vi "SW Arch draft.vi"() -> ()   [LabVIEW 2009]
panel:
  out "Main State":string
  out "VFH cluster":cluster{"VFH Message":string, "VFH Data":i32[]}={"VFH Message"="1000", "VFH Data"=[]}
  in  "Motor Message":string
  out "Sensor cluster":T1
  out "Motor Queue":refnum<queue>
  out "VFH Queue":refnum<queue>
  out "Communication Queue":refnum<queue>
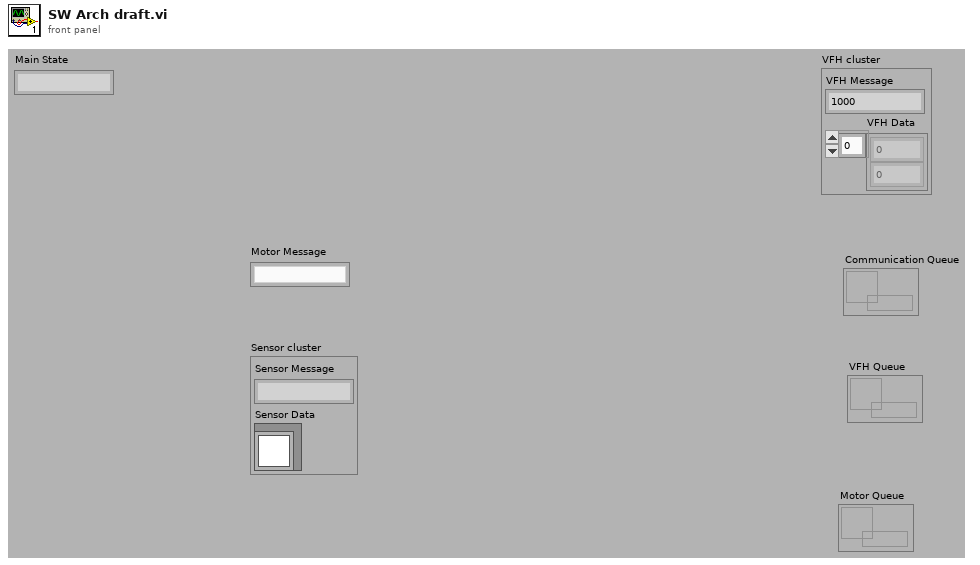
[diagram p1: front panel]
types:
  T1 = cluster{"Sensor Message":string, "Sensor Data":refnum<class>}
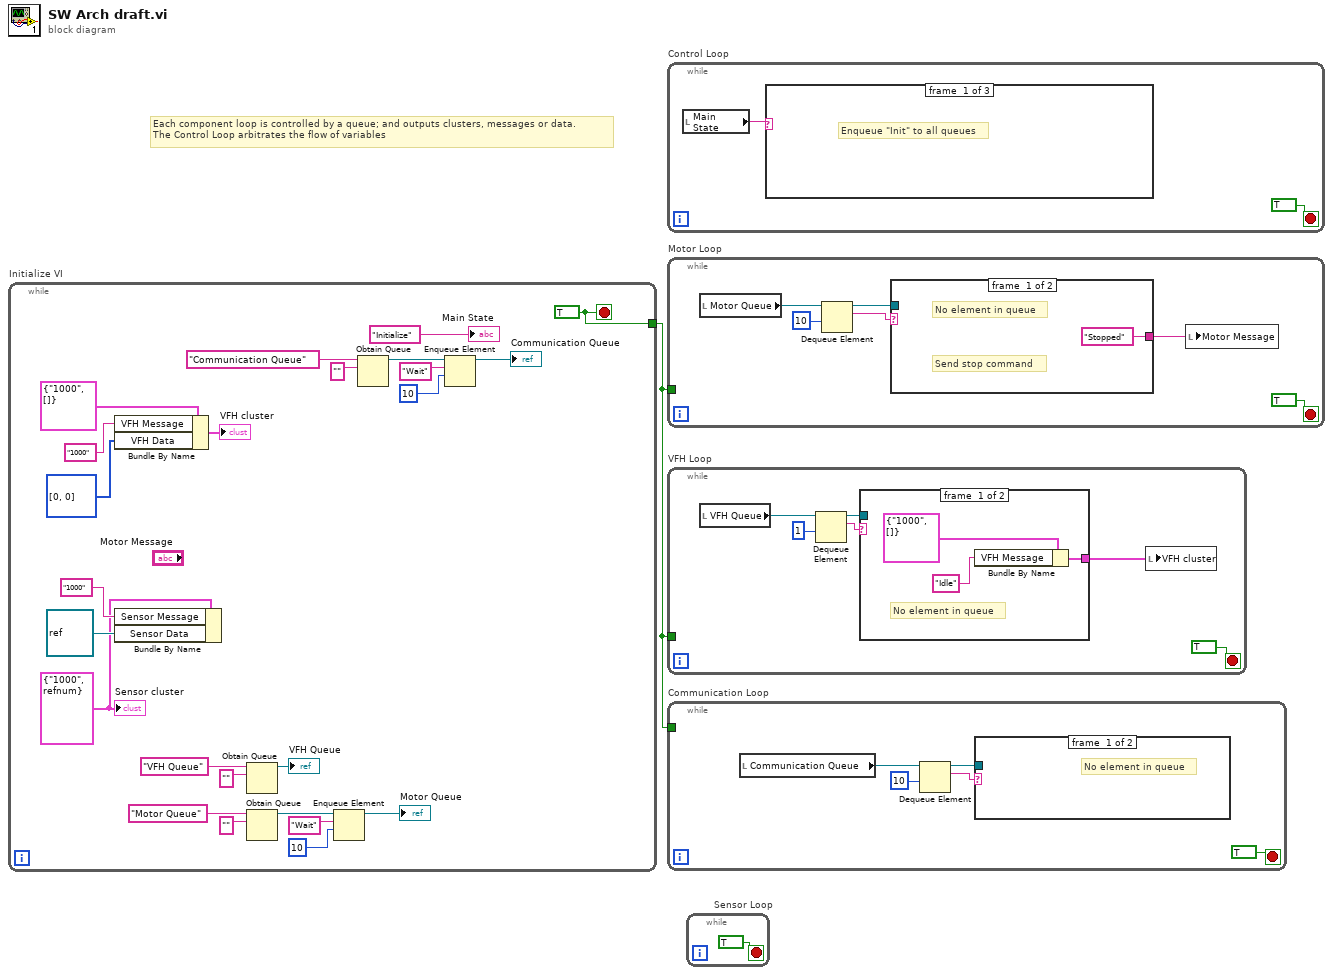
[diagram p0: block diagram]
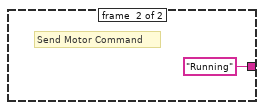
[diagram p4: hidden frame]
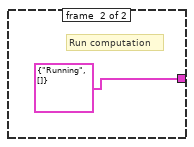
[diagram p5: hidden frame]
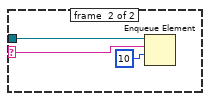
[diagram p6: hidden frame]
diagram:
  # "Each component loop is controlled by a queue; and outputs clusters, messages or data.\nThe Control Loop arbitrates the flow of variables"
  n1 = while "Initialize VI" {
    tunnel: [w10] -> w1
    stop <- w10 stop-if-true
    w5 = T1 {"Sensor Message"="1000", "Sensor Data"=refnum} ("Sensor cluster")
    w10 = TRUE
    n2 = Bundle By Name(cluster=cluster{"VFH Message":string, "VFH Data":i32[]} {"VFH Message"="1000", "VFH Data"=[]} ("VFH cluster"), "VFH Message"="1000", "VFH Data"=i32[] [0, 0]) -> (→"VFH cluster":cluster{"VFH Message":string, "VFH Data":i32[]})
    n3 = Bundle By Name(cluster=w5, "Sensor Message"="1000" ("VFH Message"), "Sensor Data"=refnum<class> refnum) -> ()  [unwired: 1 out]
    n4 = Obtain Queue(name (unnamed)="VFH Queue", element data type="" ("name (unnamed)")) -> (queue out=→"VFH Queue":refnum<queue>)  [unwired: 3 in, 2 out]
    n5 = Obtain Queue(name (unnamed)="Motor Queue", element data type="" ("name (unnamed)")) -> (queue out=w17:refnum<queue>)  [unwired: 3 in, 2 out]
    n6 = Enqueue Element(queue=w17, element="Wait", timeout in ms (-1)=10) -> (queue out=→"Motor Queue":refnum<queue>)  [unwired: 1 in, 2 out]
    n7 = Obtain Queue(name (unnamed)="Communication Queue", element data type="" ("name (unnamed)")) -> (queue out=w25:refnum<queue>)  [unwired: 3 in, 2 out]
    n8 = Enqueue Element(queue=w25, element="Wait", timeout in ms (-1)=10) -> (queue out=→"Communication Queue":refnum<queue>)  [unwired: 1 in, 2 out]
    "Sensor cluster" <- w5
    "Main State" <- "Initialize" ("Main State")
  }
  n9 = while "Control Loop" {
    stop <- TRUE stop-if-true
    n10 = local read "Main State"() -> (w26:string)
    n11 = case shown="\"RC Run\"" w26 {
      frame #0 {
        # "Enqueue \"Init\" to all queues"
      }
      frame #1 {
        # "Run Sensor\nRun VFH on new SICK data\nSensor Data -> VFH\nVFH Data -> Motor"
      }
      frame #2 {
        # "Communication Data -> Motor"
      }
    }
  }
  n12 = while "Motor Loop" {
    tunnel: w1 -> [_]
    stop <- TRUE stop-if-true
    n13 = local read "Motor Queue"() -> (w33:refnum<queue>)
    n14 = Dequeue Element(queue=w33, timeout in ms (-1)=10) -> (queue out=w30:refnum<queue>, element=w32:string)  [unwired: 1 in, 2 out]
    n15 = case shown="\"Run\"" w32 {
      tunnel: w30 -> [_ _]
      tunnel: ["Stopped" ("Motor Message") "Running" ("Motor Message")] -> w28
      frame #0 {
        # "Send stop command"
        # "No element in queue"
      }
      frame #1 {
        # "Send Motor Command"
      }
    }
    n16 = local write "Motor Message"(w28) -> ()
  }
  n17 = while "VFH Loop" {
    tunnel: w1 -> [_]
    stop <- TRUE stop-if-true
    n18 = local read "VFH Queue"() -> (w41:refnum<queue>)
    n19 = Dequeue Element(queue=w41, timeout in ms (-1)=1) -> (queue out=w38:refnum<queue>, element=w40:string)  [unwired: 1 in, 2 out]
    n20 = case shown="\"Run\"" w40 {
      tunnel: w38 -> [_ _]
      tunnel: [w44 cluster{"VFH Message":string, "VFH Data":i32[]} {"VFH Message"="Running", "VFH Data"=[]} ("VFH cluster")] -> w36
      frame #0 {
        # "No element in queue"
        n21 = Bundle By Name(cluster=cluster{"VFH Message":string, "VFH Data":i32[]} {"VFH Message"="1000", "VFH Data"=[]} ("VFH cluster"), "VFH Message"="Idle") -> (w44:cluster{"VFH Message":string, "VFH Data":i32[]})
      }
      frame #1 {
        # "Run computation"
      }
    }
    n22 = local write "VFH cluster"(w36) -> ()
  }
  n23 = while "Communication Loop" {
    tunnel: w1 -> [_]
    stop <- TRUE stop-if-true
    n24 = local read "Communication Queue"() -> (w50:refnum<queue>)
    n25 = Dequeue Element(queue=w50, timeout in ms (-1)=10) -> (queue out=w47:refnum<queue>, element=w49:string)  [unwired: 1 in, 2 out]
    n26 = case shown="\"Wait\"" w49 {
      selector: w49 -> [_ w52]
      tunnel: w47 -> [_ w53]
      frame #0 {
        # "No element in queue"
      }
      frame #1 {
        n27 = Enqueue Element(queue=w53, element=w52, timeout in ms (-1)=10) -> ()  [unwired: 1 in, 3 out]
      }
    }
  }
  n28 = while "Sensor Loop" {
    stop <- TRUE stop-if-true
  }
